vi "Get Inner Decoration.vi"() -> ()   [LabVIEW 2012] (continued)
  (unwired) 21764 items=[".NET容器"=2125, ".NET引用句柄"=3441, "10的幂"=1212, "10的自然对数"=23513, "2的幂"=1223, "2的自然对数"=23514, "ActiveX容器"=2072, "Agitator"=3831, "Array Interface Control"=23777, "Bin#1"=3073, "Bin#2"=21755, "CAN接口（程序框图常量）"=2123, "CAN接口（经典）"=3339, "CAN接口（系统）"=21964, "CAN接口（新式）"=21815, "CAN任务（程序框图常量）"=3471, "CAN任务（经典）"=3470, "CAN任务（系统）"=21963, "CAN任务（新式）"=21789, "CAN通道（程序框图常量）"=2124, "CAN通道（经典）"=3340, "CAN通道（系统）"=21966, "CAN通道（新式）"=21817, "CPU信息"=24130, "DAQmx换算名（程序框图常量）"=2116, "DAQmx换算名（经典）"=3317, "DAQmx换算名（系统）"=21952, "DAQmx换算名（新式）"=21775, "DAQmx接线端（程序框图常量）"=2117, "DAQmx接线端（经典）"=3319, "DAQmx接线端（系统）"=21955, "DAQmx接线端（新式）"=21781, "DAQmx开关（程序框图常量）"=2121, "DAQmx开关（经典）"=3337, "DAQmx开关（系统）"=21953, "DAQmx开关（新式）"=21776, "DAQmx模拟触发器源（程序框图常量）"=2119, "DAQmx模拟触发器源（经典）"=3336, "DAQmx模拟触发器源（系统）"=21951, "DAQmx模拟触发器源（新式）"=21774, "DAQmx全局通道（程序框图常量）"=3430, "DAQmx全局通道（经典）"=3443, "DAQmx全局通道（系统）"=21957, "DAQmx全局通道（新式）"=21770, "DAQmx任务名（程序框图常量）"=3434, "DAQmx任务名（经典）"=3442, "DAQmx任务名（系统）"=21959, "DAQmx任务名（新式）"=21778, "DAQmx设备名（程序框图常量）"=2093, "DAQmx设备名（经典）"=3318, "DAQmx设备名（系统）"=21950, "DAQmx设备名（新式）"=21773, "DAQmx物理通道（程序框图常量）"=2118, "DAQmx物理通道（经典）"=3335, "DAQmx物理通道（系统）"=21954, "DAQmx物理通道（新式）"=21777, "DataSocket引用句柄"=3417, "EOF"=1410, "exp(Arg)-1"=1222, "e的倒数"=23511, "FieldPoint IO点（程序框图常量）"=3440, "FieldPoint IO点（经典）"=3439, "FieldPoint IO点（新式）"=21784, "FIFO引用句柄"=3474, "For循环"=2002, "FPGA引用句柄至会话句柄转换"=2322, "Furnace"=3829, "GPIB初始化"=1957, "GPIB触发"=1953, "GPIB串行轮询"=1955, "GPIB等待"=1958, "GPIB读取"=1951, "GPIB其它命令"=1956, "GPIB清零"=1954, "GPIB写入"=1950, "GPIB状态"=1959, "IMAQ会话句柄"=3415, "IP地址至字符串转换"=1710, "IVI逻辑名称（程序框图常量）"=3420, "IVI逻辑名称（经典）"=3414, "IVI逻辑名称（新式）"=21736, "IVI删除会话句柄"=8103, "IVI新建会话句柄"=8102, "LabVIEW对象"=3457, "MathScript节点"=2357, "MATLAB脚本"=9020, "OLE变体"=3150, "Pi"=23504, "Pi乘以2"=23505, "Pi除以2"=23506, "Pi的倒数"=23507, "Pi的自然对数"=23508, "RT FIFO创建"=24000, "RT FIFO读取"=24001, "RT FIFO删除"=24003, "RT FIFO写入"=24002, "Simon量表"=32600, "Sinc"=1227, "TCP平化读取"=1718, "TCP平化写入"=1719, "TCP网络连接引用句柄"=3407, "TCP自由读取"=1720, "TCP自由写入"=1721, "TDMS Close"=24113, "TDMS Defragment"=24119, "TDMS Flush"=24117, "TDMS Get Properties"=24115, "TDMS List Contents"=24116, "TDMS Open"=24112, "TDMS Read"=24111, "TDMS Refnum To File ID"=24120, "TDMS Set Properties"=24114, "TDMS Write"=24110, "TDMS Write IP"=24118, "TDMS文件"=3477, "UDP网络连接引用句柄"=3418, "UTF-8至文本转换"=23067, "Variable Configuration"=3475, "VISA GPIB传递IFC"=2318, "VISA GPIB传递控制权"=2317, "VISA GPIB控制ATN"=2316, "VISA GPIB控制REN"=2304, "VISA GPIB命令"=2315, "VISA USB控制输出"=2087, "VISA USB控制输入"=2086, "VISA VXI命令或查询"=2305, "VISA查找资源"=1923, "VISA存数16"=1935, "VISA存数32"=1996, "VISA存数64"=2143, "VISA存数8"=1939, "VISA打开"=2308, "VISA等待事件"=1943, "VISA读取"=1925, "VISA读取STB"=1928, "VISA读取设备并写入文件"=2313, "VISA读取文件并写入设备"=2314, "VISA放弃事件"=1941, "VISA关闭"=1922, "VISA解锁"=1994, "VISA禁用事件"=1940, "VISA内存分配"=1997, "VISA内存分配Ex"=2146, "VISA内存释放"=1998, "VISA启用事件"=1942, "VISA清空I/O缓冲区"=2302, "VISA取数16"=1934, "VISA取数32"=1995, "VISA取数64"=2142, "VISA取数8"=1938, "VISA取消触发映射"=2312, "VISA取消地址映射"=1933, "VISA设备清零"=1927, "VISA设置I/O缓冲区大小"=2301, "VISA输出16"=1931, "VISA输出32"=1945, "VISA输出64"=2141, "VISA输出8"=1937, "VISA输入16"=1930, "VISA输入32"=1944, "VISA输入64"=2140, "VISA输入8"=1936, "VISA锁"=1993, "VISA写入"=1926, "VISA引用句柄至会话句柄转换"=2300, "VISA映射触发"=2311, "VISA映射地址"=1932, "VISA置触发有效"=1929, "VISA置效用信号有效"=2310, "VISA置中断信号有效"=2309, "VISA转出16"=1949, "VISA转出32"=1992, "VISA转出64"=2145, "VISA转出8"=1947, "VISA转入16"=1948, "VISA转入32"=1991, "VISA转入64"=2144, "VISA转入8"=1946, "VISA转移"=2303, "VISA状态说明"=1924, "VISA资源名称"=3421, "VISA资源名称（经典）"=3409, "VISA资源名称（新式）"=21737, "VI服务器引用"=2091, "VI库"=1425, "VI引用句柄"=3422, "While循环#1"=2003, "While循环#2"=2352, "XY图（经典）"=3500, "XY图（新式）"=21716, "X的Y次根"=23062, "X的幂"=1213, "阿伏加德罗常数(1/mol)"=23520, "按2的幂缩放"=1074, "按名称解除捆绑"=2058, "按名称捆绑"=2057, "八进制数？"=1129, "八进制字符串至数值转换"=1186, "包矩阵"=23001, "包括定点溢出状态"=5564, "保留运行类"=8018, "比特包至数组"=3135, "变量类说明符常量"=2106, "变量名称常量"=3478, "变体"=3310, "变体至平化字符串转换"=8203, "变体至数据转换"=8003, "标签（系统）"=21961, "标签（新式）"=21960, "标识符属性下拉列表"=2063, "表达式节点"=2201, "表格（经典）"=21796, "表格（系统）"=21797, "表格（新式）"=21790, "并行轮询"=1969, "并行轮询配置"=1970, "波形图（经典）"=3504, "波形图（新式）"=21703, "波形图表"=21010, "波形图表（经典）"=3501, "波形图表（新式）"=21717, "不等于0？"=1116, "不等于？"=1105, "布尔数组至数值转换"=1815, "布尔值至(0,1)转换"=1167, "步进数值控件（系统）"=21900, "彩色矩形（断开？）"=3625, "菜单下拉列表（经典）"=3018, "菜单下拉列表（新式）"=21600, "菜单引用句柄"=3413, "测试SRQ"=1986, "层叠式顺序结构"=2000, "插入菜单项"=9003, "插入式控件"=21820, "查找请求设备"=1966, "查找侦听器"=1965, "拆分按钮"=21020, "拆分路径"=1420, "拆分数字"=1170, "拆分信号"=2351, "拆分一维数组"=1908, "产生前面板活动"=1329, "产生事件发生"=1700, "产生用户定义Trace事件"=2250, "产生用户事件"=2074, "敞口槽（经典）"=3070, "敞口槽（新式）"=21751, "敞口罐（平面，经典）"=21752, "敞口罐（阴影，经典）"=3074, "乘"=1052, "乘（带错误接线端）"=3917, "程序框图禁用结构"=2054, "抽取一维数组"=2046, "初始化数组"=2053, "除"=1053, "除（带错误接线端）"=3918, "触发"=1988, "触发设备列表"=1989, "传递控制权"=1968, "传送器"=3827, "传统DAQ通道（程序框图常量）"=2085, "传统DAQ通道（经典）"=3320, "传统DAQ通道（新式）"=21733, "串行轮询所有设备"=1960, "创建TCP侦听器"=1717, "创建波形"=2066, "创建簇数组"=2047, "创建红外线侦听器"=9140, "创建矩阵"=8500, "创建蓝牙侦听器"=9151, "创建流"=23796, "创建路径"=1419, "创建数组"=2041, "创建网络流读取方端点"=23811, "创建网络流写入方端点"=23810, "创建文件夹"=8055, "创建用户事件"=2073, "垂直分隔栏"=21860, "垂直分隔栏（经典）"=21862, "垂直分隔栏（系统）"=21864, "垂直管道（平面）"=3816, "垂直管道（阴影）"=3716, "垂直滚动条"=21111, "垂直滑动杆"=3004, "垂直滑动杆（系统）"=21903, "垂直滑动杆开关（经典）"=3115, "垂直滑动杆开关（新式）"=21741, "垂直进度条（系统）"=21909, "垂直进度条（新式）"=21104, "垂直开关"=3109, "垂直刻度条"=21107, "垂直平滑盒"=3634, "垂直翘板开关"=21740, "垂直梯度矩形"=32503, "垂直梯度椭圆"=32501, "垂直梯度圆角矩形"=32506, "垂直填充滑动杆（经典）"=3009, "垂直填充滑动杆（新式）"=21014, "垂直摇杆开关（经典）"=3111, "垂直摇杆开关（新式）"=21005, "垂直直线"=3822, "垂直指针滑动杆（经典）"=3007, "垂直指针滑动杆（系统）"=21901, "垂直指针滑动杆（新式）"=21017, "从XML还原"=8401, "从流中读取单个元素"=23797, "从流中读取多个元素"=23803, "从之前设备中读取数据"=1972, "从字符串还原"=1165, "簇（经典）"=3400, "簇（新式）"=21607, "簇常量"=2071, "簇至数组转换"=1169, "错误下拉列表常量"=2039, "打开/创建/替换数据记录文件"=8054, "打开/创建/替换文件"=8050, "打开DataSocket"=1084, "打开TCP连接"=1715, "打开UDP"=1723, "打开UDP多点传送"=1727, "打开VI对象引用"=8013, "打开VI引用"=8010, "打开变量连接"=23779, "打开并验证变量连接"=23790, "打开红外线连接"=9142, "打开蓝牙连接"=9153, "打开设备"=1430, "打开文件"=1403, "打开应用程序引用"=8012, "打开自动化"=8000, "大于0？"=1117, "大于？"=1110, "大于等于0？"=1114, "大于等于？"=1103, "带边框颜色盒（经典）"=3008, "带边框颜色盒（新式）"=21019, "带标签方形按钮"=3123, "带标签矩形按钮"=3124, "带标签椭圆形按钮"=3125, "带标签圆形按钮"=3122, "带箭头线（粗）"=3631, "带箭头线（细）"=3628, "带进位的右移位"=1607, "带进位的左移位"=1606, "带阴影的椭圆"=32509, "带阴影的圆角矩形"=32508, "代码接口节点"=2050, "单按钮对话框"=1340, "单位转换"=2059, "单选按钮（经典）"=22003, "单选按钮（系统）"=22002, "单选按钮（系统） 1"=3133, "单选按钮（新式）"=22001, "弹出菜单下拉列表"=3017, "当前VI菜单栏"=9000, "当前VI路径"=1426, "当前进程ID"=24131, "倒数"=1059, "等待(ms)"=1302, "等待GPIB RQS"=1952, "等待SRQ"=1990, "等待TCP侦听器"=1712, "等待带通知器历史的多个通知"=9132, "等待带通知器历史的通知"=9131, "等待多个通知"=9106, "等待红外线侦听器"=9143, "等待活动"=1722, "等待蓝牙侦听器"=9147, "等待前面板活动"=1328, "等待事件发生"=1701, "等待通知"=9105, "等待下一个整数倍毫秒"=1327, "等于0？"=1113, "等于？"=1102, "底数为10的对数"=1210, "底数为2的对数"=1225, "底数为X的对数"=1224, "电子表格字符串至数组转换"=1539, "调用父方法"=2354, "调用节点"=3900, "调用库函数节点"=2062, "调用链"=1999, "调整矩阵大小"=8508, "定点溢出？"=5565, "定点转换为整型"=5566, "定时顺序"=5573, "定时循环"=5570, "动态FPGA接口转换"=5690, "读取DataSocket"=1086, "读取TCP数据"=1716, "读取UDP数据"=1724, "读取变量"=23781, "读取变量（超时方式）"=23786, "读取二进制文件"=8051, "读取红外线数据"=9145, "读取蓝牙数据"=9149, "读取设备"=1432, "读取数据记录文件"=8069, "读取文本文件"=8070, "读取文件"=1407, "读取状态"=1973, "队列引用句柄"=3424, "队列最前端插入元素"=9129, "对话框垂直滚动条"=21906, "对话框数值#1"=2100, "对话框数值#2"=3006, "对话框水平滚动条"=21905, "对话框字符串"=2110, "多段管道"=23780, "多列列表框（经典）"=21799, "多列列表框（系统）"=21798, "多列列表框（新式）"=21791, "多速率结构"=2199, "二维数组转置"=1902, "二维图片"=3508, "发动机（平面）"=3820, "发动机（阴影）"=3720, "发送"=1977, "发送IFC"=1980, "发送LLO"=1982, "发送命令"=1978, "发送设置"=1983, "发送数据"=1979, "发送通知"=9104, "发送至设备列表"=1981, "反馈节点"=2353, "反双曲余割"=23056, "反双曲余切"=23058, "反双曲余弦"=1218, "反双曲正割"=23057, "反双曲正切"=1219, "反双曲正弦"=1217, "反余割"=23050, "反余切"=23052, "反余弦"=1207, "反正割"=23051, "反正切"=1208, "反正切（2个输入）"=1228, "反正弦"=1206, "反转一维数组"=1900, "反转字符串"=1537, "方形按钮"=3101, "方形单选按钮"=3107, "方形灯"=3105, "方形开关按钮"=3119, "方形开关按钮（性能分析）"=3113, "方形指示灯（经典）"=3121, "方形指示灯（新式）"=21013, "访问权限"=1412, "非"=1064, "非法共享变量"=23527, "非法路径常量"=23524, "非法数字/路径/引用句柄？"=1128, "非法引用句柄常量"=23526, "分叉"=2194, "分解变体"=2404, "分解数组"=2412, "分解锁定数据变量引用"=2406, "分数/指数字符串至数值转换"=1187, "符号"=1049, "浮点数等于？"=23064, "复共轭"=1048, "复合运算"=2200, "复数至极坐标转换"=1045, "复数至实部虚部转换"=1044, "复选框（经典）"=3117, "复选框（系统）"=3132, "复选框（新式）"=21924, "复制"=8053, "复制（过时）"=1416, "负无穷大"=23509, "格式化日期/时间字符串"=8100, "格式化写入文件"=2083, "格式化写入字符串"=2081, "格式化值"=1512, "公式节点"=2004, "共享变量"=23778, "共享变量常量"=3473, "共享变量控件（经典）"=3472, "共享变量控件（新式）"=21814, "共享变量至字符串转换"=1831, "构造器节点"=3904, "关闭DataSocket"=1085, "关闭TCP连接"=1713, "关闭UDP"=1726, "关闭变量连接"=23783, "关闭红外线连接"=9144, "关闭蓝牙连接"=9148, "关闭文件"=8052, "关闭文件（过时）"=1405, "关闭引用"=8011, "关闭自动化"=8001, "合并错误"=2147, "合并信号"=2350, "红外线网络连接引用句柄"=3450, "滑动开关"=21011, "缓存级别数量"=24133, "换行符常量"=23501, "回车键常量"=23500, "回调事件引用句柄"=3435, "会话句柄至引用句柄转换"=2307, "混合复选框（系统）"=21333, "混合信号图"=21721, "获取帮助窗口状态"=1354, "获取变体属性"=8205, "获取波形成分"=2067, "获取波形属性"=8208, "获取菜单项信息"=9005, "获取定点分量"=11163, "获取队列引用"=9108, "获取队列状态"=9110, "获取记录数量"=8064, "获取矩阵对角"=8501, "获取矩阵元素"=8502, "获取卷信息"=8067, "获取快捷菜单信息"=9007, "获取权限"=8065, "获取日期/时间（秒）"=1303, "获取日期/时间字符串"=1600, "获取数据记录位置"=8061, "获取所选菜单项"=9001, "获取通知器引用"=9101, "获取通知器状态"=9103, "获取拖放数据"=9154, "获取文件大小"=8063, "获取文件类型和创建者"=8066, "获取文件位置"=8062, "获取子矩阵"=8503, "或"=1062, "或非"=1072, "基本单位转换"=1079, "极坐标至复数转换"=1047, "极坐标至实部虚部转换"=23061, "计算机ε"=23528, "加"=1050, "加1"=1057, "加（带错误接线端）"=3915, "假常量"=2006, "检查值"=3833, "简易垂直滑动杆"=3002, "简易数值"=2900, "简易水平滑动杆"=3003, "简易字符串"=2115, "减"=1051, "减1"=1058, "减（带错误接线端）"=3916, "交叉"=2197, "交换器"=3828, "交换向量元素"=1912, "交换值"=2401, "交换字"=1163, "交换字节"=1162, "交织一维数组"=2045, "接收数据"=1974, "截取字符串"=1503, "解除捆绑"=2048, "静态VI引用"=2084, "旧VISA打开"=1921, "局部变量"=2061, "矩形停止按钮"=3128, "矩阵大小"=8507, "矩阵转置"=8509, "拒绝访问"=8057, "句柄存数"=1605, "句柄取数"=1604, "卷信息"=1414, "绝对值"=1054, "开关按钮"=21001, "可打印？"=1124, "空白？"=1125, "空路径常量"=23523, "空数组？"=23063, "空字符串/路径？"=1112, "空字符串常量"=23503, "控件引用句柄"=3419, "控件与仿真循环"=2099, "控制帮助窗口"=1353, "控制在线帮助"=1355, "捆绑"=2049, "蓝牙网络连接引用句柄"=3468, "类说明符常量"=2094, "类型和创建者"=1434, "里德伯常数(1/m)"=23521, "连接"=2195, "连接字符串"=2040, "量表（经典）"=3040, "量表（新式）"=21009, "列表框（经典）"=21806, "列表框（系统）"=21805, "列表框（新式）"=21792, "列表框符号下拉列表控件常量"=2038, "列表目录"=1418, "临时目录"=1435, "漏斗#1"=21754, "漏斗#2"=3072, "路径常量"=2009, "路径类型"=1421, "路径至字符串数组转换"=1423, "路径至字符串转换"=1077, "罗列文件夹"=8083, "逻辑移位"=1081, "枚举（经典）"=3023, "枚举（系统）"=3062, "枚举（新式）"=21605, "枚举常量"=2090, "秒至日期/时间转换"=1309, "摩尔气体常数(J/(mol K))"=23522, "默认目录"=1427, "内嵌C节点"=2104, "判定范围并强制转换"=1127, "匹配模式"=1535, "匹配真/假字符串"=1533, "匹配字符串"=1532, "平方"=23059, "平方根"=1060, "平滑的椭圆"=32500, "平滑的圆角矩形"=32505, "平化至XML"=8400, "平化至字符串"=1164, "平化字符串至变体转换"=8202, "平面反向三角形"=3623, "平面方形按钮"=3103, "平面盒"=3602, "平面框"=3608, "平面右向三角形"=3621, "平面圆盒"=3611, "平面圆形"=3605, "平面圆形按钮"=3102, "平面正向三角形"=3622, "平面左向三角形"=3620, "平铺式顺序结构"=2069, "平台平面方形按钮"=3134, "普朗克常数(J/Hz)"=23516, "启用本地模式"=1963, "启用菜单跟踪"=9002, "启用远程模式"=1964, "强度图（经典）"=3510, "强度图（新式）"=21720, "强度图表（经典）"=3509, "强度图表（新式）"=21719, "强制类型转换"=1166, "强制转换至类型"=2402, "翘板开关"=21002, "清除定点溢出状态"=5562, "清空队列"=9114, "请求释放内存"=1610, "区域"=2196, "取负数"=1069, "取消按钮（系统）"=3131, "取消按钮（新式）"=21739, "取消并行轮询配置"=1971, "取消释放变体值引用"=2411, "取消通知"=9107, "取消注册会话句柄"=2320, "取消注册事件"=2076, "全局变量"=2060, "确定按钮（系统）"=3130, "确定按钮（新式）"=21738, "日期/时间至秒转换"=1308, "三维图片"=23776, "扫描变量读取"=23784, "扫描变量写入"=23787, "扫描文件"=2082, "扫描值"=1534, "扫描字符串"=2080, "删除"=8056, "删除（过时）"=1417, "删除变体属性"=8206, "删除波形属性"=8209, "删除菜单项"=9004, "删除定点溢出状态"=5563, "删除数据值引用"=2409, "删除数组元素"=3912, "商与余数"=1056, "上矩形值（轮廓）"=21762, "上矩形值（平面）"=3702, "上矩形值（阴影）"=3802, "上凸反向三角形"=3615, "上凸盒（经典）"=3600, "上凸盒（新式）"=3637, "上凸框"=3606, "上凸右向三角形"=3613, "上凸圆盒"=3609, "上凸圆形"=3603, "上凸正向三角形"=3614, "上凸左向三角形"=3612, "设备控制/状态"=1433, "设备清零"=1961, "设备清零列表"=1962, "设备引用句柄"=3405, "设置RWLS"=1984, "设置变体属性"=8204, "设置波形属性"=8207, "设置菜单项信息"=9006, "设置超时"=1985, "设置记录数量"=8075, "设置矩阵对角"=8504, "设置矩阵元素"=8505, "设置句柄大小"=1603, "设置权限"=8076, "设置事件发生"=1702, "设置数据记录位置"=8072, "设置文件大小"=8074, "设置文件类型和创建者"=8077, "设置文件位置"=8073, "设置子矩阵"=8506, "生成地址"=1967, "十进制数？"=1119, "十进制数字符串至数值转换"=1184, "十六进制数？"=1123, "十六进制数字符串至数值转换"=1185, "时间标识（程序框图常量）"=2068, "时间标识输入控件（经典）"=5555, "时间标识输入控件（系统）"=21967, "时间标识输入控件（新式）"=21913, "时间标识显示控件（经典）"=5556, "时间标识显示控件（新式）"=21914, "时间计数器"=1300, "实部虚部至复数转换"=1046, "实部虚部至极坐标转换"=23060, "事件发生引用句柄"=3406, "事件回调注册"=2078, "事件结构"=2052, "事件数据节点"=2102, "释放变体值引用"=2410, "释放队列引用"=9109, "释放通知器引用"=9102, "首次调用？"=1083, "属性节点"=1920, "树形控件（经典）"=21819, "树形控件（系统）"=21794, "树形控件（新式）"=21793, "数据缓冲区大小"=24132, "数据记录文件引用句柄"=3402, "数据值引用"=3476, "数据值引用常量"=24134, "数值常量"=2005, "数值控件（经典）"=3000, "数值控件（系统）"=21919, "数值控件（新式）"=21003, "数值显示控件（经典）"=3001, "数值显示控件（新式）"=21004, "数值至八进制字符串转换"=1182, "数值至布尔数组转换"=1814, "数值至工程字符串转换"=1183, "数值至十进制数字符串转换"=1180, "数值至十六进制字符串转换"=1181, "数值至小数字符串转换"=1506, "数值至指数字符串转换"=1505, "数字波形图（经典）"=3511, "数字波形图（新式）"=21718, "数字数据（经典）"=3210, "数字数据（新式）"=21216, "数组（程序框图常量）"=2070, "数组（经典）"=3300, "数组（新式）"=21608, "数组插入"=3911, "数组大小"=1809, "数组元素或操作"=1910, "数组元素相乘"=1904, "数组元素相加"=1903, "数组元素与操作"=1911, "数组至比特包"=3136, "数组至簇转换"=1168, "数组至电子表格字符串转换"=1540, "数组子集"=2044, "数组最大值与最小值"=1907, "刷新流"=23808, "刷新文件"=8059, "刷新文件（过时）"=1406, "双按钮对话框"=1341, "双曲余割"=23053, "双曲余切"=23055, "双曲余弦"=1215, "双曲正割"=23054, "双曲正切"=1216, "双曲正弦"=1214, "水平按钮框"=3636, "水平分隔栏"=21861, "水平分隔栏（经典）"=21863, "水平分隔栏（系统）"=21865, "水平管道（平面）"=3810, "水平管道（阴影）"=3710, "水平罐"=3071, "水平滚动条"=21110, "水平滑动杆（经典）"=3010, "水平滑动杆（系统）"=21904, "水平滑动开关"=3114, "水平进度条（系统）"=21910, "水平进度条（新式）"=21102, "水平开关"=3108, "水平刻度条"=21106, "水平平滑盒"=3633, "水平梯度矩形"=32504, "水平梯度椭圆"=32502, "水平梯度圆角矩形"=32507, "水平填充滑动杆（经典）"=3012, "水平填充滑动杆（新式）"=21100, "水平线"=3821, "水平摇杆开关（经典）"=3110, "水平摇杆开关（新式）"=21700, "水平指针滑动杆（经典）"=3011, "水平指针滑动杆（系统）"=21902, "水平指针滑动杆（新式）"=21101, "搜索"=1409, "搜索/拆分字符串"=1538, "搜索变量容器"=23802, "搜索红外线"=9141, "搜索蓝牙设备"=9152, "搜索替换字符串"=3914, "搜索一维数组"=1901, "随机数(0-1)"=1070, "索引数组"=2042, "索引与捆绑簇数组"=2056, "索引字符串数组"=1531, "锁定范围"=1411, "替换数组子集"=3910, "替换子字符串"=3913, "添加真/假字符串"=1511, "条件结构"=2001, "条件禁用结构"=2064, "停止"=1350, "停止按钮"=21230, "通过引用调用"=3901, "通过引用调用MathScript"=3906, "通知器引用句柄"=3423, "同或"=1073, "图片下拉列表（经典）"=3015, "图片下拉列表（系统）"=21925, "图片下拉列表（新式）"=21602, "退出LabVIEW"=1352, "尾数与指数"=1150, "未组合的矩阵"=23000, "温度计（经典）"=3021, "温度计（新式）"=21007, "文本按钮"=21015, "文本下拉列表（程序框图常量）"=2008, "文本下拉列表（经典）"=3014, "文本下拉列表（系统）"=3060, "文本下拉列表（新式）"=21601, "文本与图片下拉列表（经典）"=3016, "文本与图片下拉列表（新式）"=21603, "文本至UTF-8转换"=23066, "文件/目录信息"=8082, "文件/目录信息（过时）"=1413, "文件对话框"=8058, "文件对话框（过时）"=8081, "文件路径输入控件（经典）"=3203, "文件路径输入控件（系统）"=21922, "文件路径输入控件（新式）"=21730, "文件路径显示控件（经典）"=3204, "文件路径显示控件（新式）"=21731, "系统测试"=1987, "系统复位"=1976, "下凹菜单下拉列表"=3019, "下凹反向三角形"=3619, "下凹盒"=3601, "下凹盒（粗）"=3635, "下凹框（系统）"=3624, "下凹框（新式）"=3607, "下凹右向三角形"=3617, "下凹圆盒"=3610, "下凹圆盒 1"=3638, "下凹圆形"=3604, "下凹正向三角形"=3618, "下凹左向三角形"=3616, "下矩形值（轮廓）"=3806, "下矩形值（平面）"=3706, "下矩形值（阴影）"=21766, "下拉菜单下拉列表"=3061, "线条（粗）"=3629, "线条（分隔，粗）"=3630, "线条（分隔，系统）"=3632, "线条（分隔，细）"=3627, "线条（细）"=3626, "像素图"=3505, "像素图（警告：危险）"=3507, "向流中写入单个元素"=23798, "向流中写入多个元素"=23804, "向上T形（平面）"=3812, "向上T形（阴影）"=3712, "向上箭头"=3823, "向上箭头值（轮廓）"=3803, "向上箭头值（平面）"=3703, "向上箭头值（阴影）"=21763, "向上取整"=1076, "向下T形（平面）"=3818, "向下T形（阴影）"=3718, "向下箭头"=3824, "向下箭头值（轮廓）"=3807, "向下箭头值（平面）"=3707, "向下箭头值（阴影）"=21767, "向下取整"=1075, "向右T形（平面）"=3815, "向右T形（阴影）"=3715, "向左T形（平面）"=3809, "向左T形（阴影）"=3709, "向左箭头值（轮廓）"=3801, "向左箭头值（平面）"=3701, "向左箭头值（阴影）"=21761, "销毁流端点"=23794, "销毁用户事件"=2075, "小于0？"=1118, "小于？"=1111, "小于等于0？"=1115, "小于等于？"=1104, "写入DataSocket"=1087, "写入TCP数据"=1714, "写入UDP数据"=1725, "写入变量"=23782, "写入变量（超时方式）"=23789, "写入二进制文件"=8078, "写入红外线数据"=9146, "写入蓝牙数据"=9150, "写入设备"=1431, "写入数据记录文件"=8079, "写入文本文件"=8080, "写入文件"=1408, "新建VI"=8014, "新建VI对象"=8015, "新建目录"=1402, "新建数据值引用"=2408, "新文件"=1404, "行结束常量"=23525, "旋钮（经典）"=3005, "旋钮（新式）"=21000, "旋转供给器"=3830, "选项卡控件（经典）"=3330, "选项卡控件（系统）"=3331, "选项卡控件（新式）"=3332, "选行并添加至字符串"=1510, "选择"=1516, "循环移位"=1082, "压力罐（平面）"=3075, "压力罐（阴影）"=21753, "压缩器"=3832, "颜色盒"=3013, "颜色盒常量"=2120, "颜色盒窄边"=2905, "颜色梯度"=3022, "液罐（经典）"=3020, "液罐（新式）"=21006, "一维数组插值"=1905, "一维数组排序"=1120, "一维数组循环移位"=1906, "一维数组转置"=23068, "移动"=8068, "移动（过时）"=1415, "仪表（经典）"=3030, "仪表（新式）"=21008, "以10为底的e的对数"=23512, "以阈值插值一维数组"=1909, "异或"=1063, "引用句柄至会话句柄转换"=2306, "引用句柄至路径转换"=1424, "应用程序引用句柄"=3412, "用户定义标识符（程序框图常量）"=2114, "用户定义标识符（经典）"=3329, "用户定义标识符（新式）"=21749, "用户定义引用句柄"=3428, "用户定义引用句柄标识符（程序框图常量）"=3426, "用户定义引用句柄标识符（经典）"=3429, "用户定义引用句柄标识符（新式）"=21745, "用户定义引用句柄标识符平化（经典）"=3454, "用户定义引用句柄标识符平化（新式）"=21747, "用户项"=3506, "有损耗元素入队列"=9130, "右泵（平面）"=3819, "右泵（阴影）"=3719, "右箭头"=3825, "右箭头值（轮廓）"=3805, "右箭头值（平面）"=3705, "右箭头值（阴影）"=21765, "右矩形值（轮廓）"=3804, "右矩形值（平面）"=3704, "右矩形值（阴影）"=21764, "右上弯管（平面）"=3814, "右上弯管（阴影）"=3714, "右下弯管（平面）"=3817, "右下弯管（阴影）"=3717, "余割"=1204, "余切"=1205, "余弦"=1201, "与"=1061, "与非"=1071, "预分配的读取二进制文件"=24135, "预览队列元素"=9112, "元电荷(C)"=23517, "元素出队列"=9113, "元素入队列"=9111, "元素同址操作结构"=2360, "圆形按钮"=3100, "圆形单选按钮"=3106, "圆形灯"=3104, "圆形开关按钮"=3118, "圆形开关按钮（性能分析）"=3112, "圆形停止按钮"=3127, "圆形指示灯（经典）"=3120, "圆形指示灯（新式）"=21012, "运动资源（程序框图常量）"=3449, "运动资源（经典）"=3448, "运动资源（新式）"=21787, "蕴含"=1080, "在后台打开变量连接"=23791, "在字符串中搜索标记"=8101, "真空光速(m/sec)"=23518, "整数拼接"=1171, "整型转换为定点"=5567, "正割"=1203, "正切"=1202, "正无穷大"=23515, "正弦"=1200, "正弦与余弦"=1220, "直接变量读取"=23785, "直接变量写入"=23788, "指示灯按钮"=3116, "指数"=1211, "制表符常量"=23502, "重力常数(Nm2/kg2)"=23519, "重排数组维数"=2055, "重组变体（警告：危险）"=2405, "重组解锁数据变量引用（警告：危险）"=2407, "重组数组"=2403, "注册会话句柄"=2319, "注册事件"=2065, "转换为64位整型"=1155, "转换为OLE变体"=8002, "转换为变体"=8201, "转换为长整型"=1142, "转换为大写字母"=1188, "转换为单精度浮点数"=1146, "转换为单精度复数"=1151, "转换为单字节整型"=1140, "转换为定点数"=5561, "转换为扩展精度浮点数"=1149, "转换为扩展精度复数"=1154, "转换为时间标识"=5560, "转换为双精度浮点数"=1147, "转换为双精度复数"=1152, "转换为双字节整型"=1141, "转换为探针字符串"=2413, "转换为特定的类"=8016, "转换为通用的类"=8017, "转换为无符号64位整型"=1156, "转换为无符号长整型"=1145, "转换为无符号单字节整型"=1143, "转换为无符号双字节整型"=1144, "转换为小写字母"=1189, "转盘（经典）"=3050, "转盘（新式）"=21732, "状态"=2198, "状态图"=2051, "准备接收"=1975, "资源索引"=1088, "子面板"=21810, "子面板（经典）"=21811, "子面板（系统）"=21823, "自动化引用句柄"=3410, "自然对数"=1209, "自然对数 (Arg +1)"=1221, "自然对数的底数"=23510, "自由标签"=2321, "字符串常量"=2007, "字符串长度"=1502, "字符串输入控件（经典）"=3200, "字符串输入控件（系统）"=21920, "字符串输入控件（新式）"=21701, "字符串数组排序"=23065, "字符串数组至路径转换"=1422, "字符串显示控件（经典）"=3201, "字符串显示控件（新式）"=21702, "字符串移位"=1536, "字符串至IP地址转换"=1711, "字符串至共享变量转换"=1830, "字符串至路径转换"=1078, "字符串至字节数组转换"=1608, "字符类"=1126, "字节流文件引用句柄"=3408, "字节数组至字符串转换"=1609, "总是复制"=2400, "组合框（经典）"=3304, "组合框（系统）"=21917, "组合框（新式）"=21604, "组合框常量"=2088, "最大值与最小值"=1108, "最近数取整"=1055, "左泵（平面）"=3813, "左泵（阴影）"=3713, "左箭头"=3826, "左矩形值（轮廓）"=3800, "左矩形值（平面）"=3700, "左矩形值（阴影）"=21760, "左上弯管（平面）"=3808, "左上弯管（阴影）"=3708, "左下弯管（平面）"=3811, "左下弯管（阴影）"=3711]
  (unwired) 21764 items=[".NET容器"=2125, ".NET引用句柄"=3441, "10的幂"=1212, "10的自然对数"=23513, "2的幂"=1223, "2的自然对数"=23514, "ActiveX容器"=2072, "Agitator"=3831, "Array Interface Control"=23777, "Bin#1"=3073, "Bin#2"=21755, "CAN接口（程序框图常量）"=2123, "CAN接口（经典）"=3339, "CAN接口（系统）"=21964, "CAN接口（新式）"=21815, "CAN任务（程序框图常量）"=3471, "CAN任务（经典）"=3470, "CAN任务（系统）"=21963, "CAN任务（新式）"=21789, "CAN通道（程序框图常量）"=2124, "CAN通道（经典）"=3340, "CAN通道（系统）"=21966, "CAN通道（新式）"=21817, "CPU信息"=24130, "DAQmx换算名（程序框图常量）"=2116, "DAQmx换算名（经典）"=3317, "DAQmx换算名（系统）"=21952, "DAQmx换算名（新式）"=21775, "DAQmx接线端（程序框图常量）"=2117, "DAQmx接线端（经典）"=3319, "DAQmx接线端（系统）"=21955, "DAQmx接线端（新式）"=21781, "DAQmx开关（程序框图常量）"=2121, "DAQmx开关（经典）"=3337, "DAQmx开关（系统）"=21953, "DAQmx开关（新式）"=21776, "DAQmx模拟触发器源（程序框图常量）"=2119, "DAQmx模拟触发器源（经典）"=3336, "DAQmx模拟触发器源（系统）"=21951, "DAQmx模拟触发器源（新式）"=21774, "DAQmx全局通道（程序框图常量）"=3430, "DAQmx全局通道（经典）"=3443, "DAQmx全局通道（系统）"=21957, "DAQmx全局通道（新式）"=21770, "DAQmx任务名（程序框图常量）"=3434, "DAQmx任务名（经典）"=3442, "DAQmx任务名（系统）"=21959, "DAQmx任务名（新式）"=21778, "DAQmx设备名（程序框图常量）"=2093, "DAQmx设备名（经典）"=3318, "DAQmx设备名（系统）"=21950, "DAQmx设备名（新式）"=21773, "DAQmx物理通道（程序框图常量）"=2118, "DAQmx物理通道（经典）"=3335, "DAQmx物理通道（系统）"=21954, "DAQmx物理通道（新式）"=21777, "DataSocket引用句柄"=3417, "EOF"=1410, "exp(Arg)-1"=1222, "e的倒数"=23511, "FieldPoint IO点（程序框图常量）"=3440, "FieldPoint IO点（经典）"=3439, "FieldPoint IO点（新式）"=21784, "FIFO引用句柄"=3474, "For循环"=2002, "FPGA引用句柄至会话句柄转换"=2322, "Furnace"=3829, "GPIB初始化"=1957, "GPIB触发"=1953, "GPIB串行轮询"=1955, "GPIB等待"=1958, "GPIB读取"=1951, "GPIB其它命令"=1956, "GPIB清零"=1954, "GPIB写入"=1950, "GPIB状态"=1959, "IMAQ会话句柄"=3415, "IP地址至字符串转换"=1710, "IVI逻辑名称（程序框图常量）"=3420, "IVI逻辑名称（经典）"=3414, "IVI逻辑名称（新式）"=21736, "IVI删除会话句柄"=8103, "IVI新建会话句柄"=8102, "LabVIEW对象"=3457, "MathScript节点"=2357, "MATLAB脚本"=9020, "OLE变体"=3150, "Pi"=23504, "Pi乘以2"=23505, "Pi除以2"=23506, "Pi的倒数"=23507, "Pi的自然对数"=23508, "RT FIFO创建"=24000, "RT FIFO读取"=24001, "RT FIFO删除"=24003, "RT FIFO写入"=24002, "Simon量表"=32600, "Sinc"=1227, "TCP平化读取"=1718, "TCP平化写入"=1719, "TCP网络连接引用句柄"=3407, "TCP自由读取"=1720, "TCP自由写入"=1721, "TDMS Close"=24113, "TDMS Defragment"=24119, "TDMS Flush"=24117, "TDMS Get Properties"=24115, "TDMS List Contents"=24116, "TDMS Open"=24112, "TDMS Read"=24111, "TDMS Refnum To File ID"=24120, "TDMS Set Properties"=24114, "TDMS Write"=24110, "TDMS Write IP"=24118, "TDMS文件"=3477, "UDP网络连接引用句柄"=3418, "UTF-8至文本转换"=23067, "Variable Configuration"=3475, "VISA GPIB传递IFC"=2318, "VISA GPIB传递控制权"=2317, "VISA GPIB控制ATN"=2316, "VISA GPIB控制REN"=2304, "VISA GPIB命令"=2315, "VISA USB控制输出"=2087, "VISA USB控制输入"=2086, "VISA VXI命令或查询"=2305, "VISA查找资源"=1923, "VISA存数16"=1935, "VISA存数32"=1996, "VISA存数64"=2143, "VISA存数8"=1939, "VISA打开"=2308, "VISA等待事件"=1943, "VISA读取"=1925, "VISA读取STB"=1928, "VISA读取设备并写入文件"=2313, "VISA读取文件并写入设备"=2314, "VISA放弃事件"=1941, "VISA关闭"=1922, "VISA解锁"=1994, "VISA禁用事件"=1940, "VISA内存分配"=1997, "VISA内存分配Ex"=2146, "VISA内存释放"=1998, "VISA启用事件"=1942, "VISA清空I/O缓冲区"=2302, "VISA取数16"=1934, "VISA取数32"=1995, "VISA取数64"=2142, "VISA取数8"=1938, "VISA取消触发映射"=2312, "VISA取消地址映射"=1933, "VISA设备清零"=1927, "VISA设置I/O缓冲区大小"=2301, "VISA输出16"=1931, "VISA输出32"=1945, "VISA输出64"=2141, "VISA输出8"=1937, "VISA输入16"=1930, "VISA输入32"=1944, "VISA输入64"=2140, "VISA输入8"=1936, "VISA锁"=1993, "VISA写入"=1926, "VISA引用句柄至会话句柄转换"=2300, "VISA映射触发"=2311, "VISA映射地址"=1932, "VISA置触发有效"=1929, "VISA置效用信号有效"=2310, "VISA置中断信号有效"=2309, "VISA转出16"=1949, "VISA转出32"=1992, "VISA转出64"=2145, "VISA转出8"=1947, "VISA转入16"=1948, "VISA转入32"=1991, "VISA转入64"=2144, "VISA转入8"=1946, "VISA转移"=2303, "VISA状态说明"=1924, "VISA资源名称"=3421, "VISA资源名称（经典）"=3409, "VISA资源名称（新式）"=21737, "VI服务器引用"=2091, "VI库"=1425, "VI引用句柄"=3422, "While循环#1"=2003, "While循环#2"=2352, "XY图（经典）"=3500, "XY图（新式）"=21716, "X的Y次根"=23062, "X的幂"=1213, "阿伏加德罗常数(1/mol)"=23520, "按2的幂缩放"=1074, "按名称解除捆绑"=2058, "按名称捆绑"=2057, "八进制数？"=1129, "八进制字符串至数值转换"=1186, "包矩阵"=23001, "包括定点溢出状态"=5564, "保留运行类"=8018, "比特包至数组"=3135, "变量类说明符常量"=2106, "变量名称常量"=3478, "变体"=3310, "变体至平化字符串转换"=8203, "变体至数据转换"=8003, "标签（系统）"=21961, "标签（新式）"=21960, "标识符属性下拉列表"=2063, "表达式节点"=2201, "表格（经典）"=21796, "表格（系统）"=21797, "表格（新式）"=21790, "并行轮询"=1969, "并行轮询配置"=1970, "波形图（经典）"=3504, "波形图（新式）"=21703, "波形图表"=21010, "波形图表（经典）"=3501, "波形图表（新式）"=21717, "不等于0？"=1116, "不等于？"=1105, "布尔数组至数值转换"=1815, "布尔值至(0,1)转换"=1167, "步进数值控件（系统）"=21900, "彩色矩形（断开？）"=3625, "菜单下拉列表（经典）"=3018, "菜单下拉列表（新式）"=21600, "菜单引用句柄"=3413, "测试SRQ"=1986, "层叠式顺序结构"=2000, "插入菜单项"=9003, "插入式控件"=21820, "查找请求设备"=1966, "查找侦听器"=1965, "拆分按钮"=21020, "拆分路径"=1420, "拆分数字"=1170, "拆分信号"=2351, "拆分一维数组"=1908, "产生前面板活动"=1329, "产生事件发生"=1700, "产生用户定义Trace事件"=2250, "产生用户事件"=2074, "敞口槽（经典）"=3070, "敞口槽（新式）"=21751, "敞口罐（平面，经典）"=21752, "敞口罐（阴影，经典）"=3074, "乘"=1052, "乘（带错误接线端）"=3917, "程序框图禁用结构"=2054, "抽取一维数组"=2046, "初始化数组"=2053, "除"=1053, "除（带错误接线端）"=3918, "触发"=1988, "触发设备列表"=1989, "传递控制权"=1968, "传送器"=3827, "传统DAQ通道（程序框图常量）"=2085, "传统DAQ通道（经典）"=3320, "传统DAQ通道（新式）"=21733, "串行轮询所有设备"=1960, "创建TCP侦听器"=1717, "创建波形"=2066, "创建簇数组"=2047, "创建红外线侦听器"=9140, "创建矩阵"=8500, "创建蓝牙侦听器"=9151, "创建流"=23796, "创建路径"=1419, "创建数组"=2041, "创建网络流读取方端点"=23811, "创建网络流写入方端点"=23810, "创建文件夹"=8055, "创建用户事件"=2073, "垂直分隔栏"=21860, "垂直分隔栏（经典）"=21862, "垂直分隔栏（系统）"=21864, "垂直管道（平面）"=3816, "垂直管道（阴影）"=3716, "垂直滚动条"=21111, "垂直滑动杆"=3004, "垂直滑动杆（系统）"=21903, "垂直滑动杆开关（经典）"=3115, "垂直滑动杆开关（新式）"=21741, "垂直进度条（系统）"=21909, "垂直进度条（新式）"=21104, "垂直开关"=3109, "垂直刻度条"=21107, "垂直平滑盒"=3634, "垂直翘板开关"=21740, "垂直梯度矩形"=32503, "垂直梯度椭圆"=32501, "垂直梯度圆角矩形"=32506, "垂直填充滑动杆（经典）"=3009, "垂直填充滑动杆（新式）"=21014, "垂直摇杆开关（经典）"=3111, "垂直摇杆开关（新式）"=21005, "垂直直线"=3822, "垂直指针滑动杆（经典）"=3007, "垂直指针滑动杆（系统）"=21901, "垂直指针滑动杆（新式）"=21017, "从XML还原"=8401, "从流中读取单个元素"=23797, "从流中读取多个元素"=23803, "从之前设备中读取数据"=1972, "从字符串还原"=1165, "簇（经典）"=3400, "簇（新式）"=21607, "簇常量"=2071, "簇至数组转换"=1169, "错误下拉列表常量"=2039, "打开/创建/替换数据记录文件"=8054, "打开/创建/替换文件"=8050, "打开DataSocket"=1084, "打开TCP连接"=1715, "打开UDP"=1723, "打开UDP多点传送"=1727, "打开VI对象引用"=8013, "打开VI引用"=8010, "打开变量连接"=23779, "打开并验证变量连接"=23790, "打开红外线连接"=9142, "打开蓝牙连接"=9153, "打开设备"=1430, "打开文件"=1403, "打开应用程序引用"=8012, "打开自动化"=8000, "大于0？"=1117, "大于？"=1110, "大于等于0？"=1114, "大于等于？"=1103, "带边框颜色盒（经典）"=3008, "带边框颜色盒（新式）"=21019, "带标签方形按钮"=3123, "带标签矩形按钮"=3124, "带标签椭圆形按钮"=3125, "带标签圆形按钮"=3122, "带箭头线（粗）"=3631, "带箭头线（细）"=3628, "带进位的右移位"=1607, "带进位的左移位"=1606, "带阴影的椭圆"=32509, "带阴影的圆角矩形"=32508, "代码接口节点"=2050, "单按钮对话框"=1340, "单位转换"=2059, "单选按钮（经典）"=22003, "单选按钮（系统）"=22002, "单选按钮（系统） 1"=3133, "单选按钮（新式）"=22001, "弹出菜单下拉列表"=3017, "当前VI菜单栏"=9000, "当前VI路径"=1426, "当前进程ID"=24131, "倒数"=1059, "等待(ms)"=1302, "等待GPIB RQS"=1952, "等待SRQ"=1990, "等待TCP侦听器"=1712, "等待带通知器历史的多个通知"=9132, "等待带通知器历史的通知"=9131, "等待多个通知"=9106, "等待红外线侦听器"=9143, "等待活动"=1722, "等待蓝牙侦听器"=9147, "等待前面板活动"=1328, "等待事件发生"=1701, "等待通知"=9105, "等待下一个整数倍毫秒"=1327, "等于0？"=1113, "等于？"=1102, "底数为10的对数"=1210, "底数为2的对数"=1225, "底数为X的对数"=1224, "电子表格字符串至数组转换"=1539, "调用父方法"=2354, "调用节点"=3900, "调用库函数节点"=2062, "调用链"=1999, "调整矩阵大小"=8508, "定点溢出？"=5565, "定点转换为整型"=5566, "定时顺序"=5573, "定时循环"=5570, "动态FPGA接口转换"=5690, "读取DataSocket"=1086, "读取TCP数据"=1716, "读取UDP数据"=1724, "读取变量"=23781, "读取变量（超时方式）"=23786, "读取二进制文件"=8051, "读取红外线数据"=9145, "读取蓝牙数据"=9149, "读取设备"=1432, "读取数据记录文件"=8069, "读取文本文件"=8070, "读取文件"=1407, "读取状态"=1973, "队列引用句柄"=3424, "队列最前端插入元素"=9129, "对话框垂直滚动条"=21906, "对话框数值#1"=2100, "对话框数值#2"=3006, "对话框水平滚动条"=21905, "对话框字符串"=2110, "多段管道"=23780, "多列列表框（经典）"=21799, "多列列表框（系统）"=21798, "多列列表框（新式）"=21791, "多速率结构"=2199, "二维数组转置"=1902, "二维图片"=3508, "发动机（平面）"=3820, "发动机（阴影）"=3720, "发送"=1977, "发送IFC"=1980, "发送LLO"=1982, "发送命令"=1978, "发送设置"=1983, "发送数据"=1979, "发送通知"=9104, "发送至设备列表"=1981, "反馈节点"=2353, "反双曲余割"=23056, "反双曲余切"=23058, "反双曲余弦"=1218, "反双曲正割"=23057, "反双曲正切"=1219, "反双曲正弦"=1217, "反余割"=23050, "反余切"=23052, "反余弦"=1207, "反正割"=23051, "反正切"=1208, "反正切（2个输入）"=1228, "反正弦"=1206, "反转一维数组"=1900, "反转字符串"=1537, "方形按钮"=3101, "方形单选按钮"=3107, "方形灯"=3105, "方形开关按钮"=3119, "方形开关按钮（性能分析）"=3113, "方形指示灯（经典）"=3121, "方形指示灯（新式）"=21013, "访问权限"=1412, "非"=1064, "非法共享变量"=23527, "非法路径常量"=23524, "非法数字/路径/引用句柄？"=1128, "非法引用句柄常量"=23526, "分叉"=2194, "分解变体"=2404, "分解数组"=2412, "分解锁定数据变量引用"=2406, "分数/指数字符串至数值转换"=1187, "符号"=1049, "浮点数等于？"=23064, "复共轭"=1048, "复合运算"=2200, "复数至极坐标转换"=1045, "复数至实部虚部转换"=1044, "复选框（经典）"=3117, "复选框（系统）"=3132, "复选框（新式）"=21924, "复制"=8053, "复制（过时）"=1416, "负无穷大"=23509, "格式化日期/时间字符串"=8100, "格式化写入文件"=2083, "格式化写入字符串"=2081, "格式化值"=1512, "公式节点"=2004, "共享变量"=23778, "共享变量常量"=3473, "共享变量控件（经典）"=3472, "共享变量控件（新式）"=21814, "共享变量至字符串转换"=1831, "构造器节点"=3904, "关闭DataSocket"=1085, "关闭TCP连接"=1713, "关闭UDP"=1726, "关闭变量连接"=23783, "关闭红外线连接"=9144, "关闭蓝牙连接"=9148, "关闭文件"=8052, "关闭文件（过时）"=1405, "关闭引用"=8011, "关闭自动化"=8001, "合并错误"=2147, "合并信号"=2350, "红外线网络连接引用句柄"=3450, "滑动开关"=21011, "缓存级别数量"=24133, "换行符常量"=23501, "回车键常量"=23500, "回调事件引用句柄"=3435, "会话句柄至引用句柄转换"=2307, "混合复选框（系统）"=21333, "混合信号图"=21721, "获取帮助窗口状态"=1354, "获取变体属性"=8205, "获取波形成分"=2067, "获取波形属性"=8208, "获取菜单项信息"=9005, "获取定点分量"=11163, "获取队列引用"=9108, "获取队列状态"=9110, "获取记录数量"=8064, "获取矩阵对角"=8501, "获取矩阵元素"=8502, "获取卷信息"=8067, "获取快捷菜单信息"=9007, "获取权限"=8065, "获取日期/时间（秒）"=1303, "获取日期/时间字符串"=1600, "获取数据记录位置"=8061, "获取所选菜单项"=9001, "获取通知器引用"=9101, "获取通知器状态"=9103, "获取拖放数据"=9154, "获取文件大小"=8063, "获取文件类型和创建者"=8066, "获取文件位置"=8062, "获取子矩阵"=8503, "或"=1062, "或非"=1072, "基本单位转换"=1079, "极坐标至复数转换"=1047, "极坐标至实部虚部转换"=23061, "计算机ε"=23528, "加"=1050, "加1"=1057, "加（带错误接线端）"=3915, "假常量"=2006, "检查值"=3833, "简易垂直滑动杆"=3002, "简易数值"=2900, "简易水平滑动杆"=3003, "简易字符串"=2115, "减"=1051, "减1"=1058, "减（带错误接线端）"=3916, "交叉"=2197, "交换器"=3828, "交换向量元素"=1912, "交换值"=2401, "交换字"=1163, "交换字节"=1162, "交织一维数组"=2045, "接收数据"=1974, "截取字符串"=1503, "解除捆绑"=2048, "静态VI引用"=2084, "旧VISA打开"=1921, "局部变量"=2061, "矩形停止按钮"=3128, "矩阵大小"=8507, "矩阵转置"=8509, "拒绝访问"=8057, "句柄存数"=1605, "句柄取数"=1604, "卷信息"=1414, "绝对值"=1054, "开关按钮"=21001, "可打印？"=1124, "空白？"=1125, "空路径常量"=23523, "空数组？"=23063, "空字符串/路径？"=1112, "空字符串常量"=23503, "控件引用句柄"=3419, "控件与仿真循环"=2099, "控制帮助窗口"=1353, "控制在线帮助"=1355, "捆绑"=2049, "蓝牙网络连接引用句柄"=3468, "类说明符常量"=2094, "类型和创建者"=1434, "里德伯常数(1/m)"=23521, "连接"=2195, "连接字符串"=2040, "量表（经典）"=3040, "量表（新式）"=21009, "列表框（经典）"=21806, "列表框（系统）"=21805, "列表框（新式）"=21792, "列表框符号下拉列表控件常量"=2038, "列表目录"=1418, "临时目录"=1435, "漏斗#1"=21754, "漏斗#2"=3072, "路径常量"=2009, "路径类型"=1421, "路径至字符串数组转换"=1423, "路径至字符串转换"=1077, "罗列文件夹"=8083, "逻辑移位"=1081, "枚举（经典）"=3023, "枚举（系统）"=3062, "枚举（新式）"=21605, "枚举常量"=2090, "秒至日期/时间转换"=1309, "摩尔气体常数(J/(mol K))"=23522, "默认目录"=1427, "内嵌C节点"=2104, "判定范围并强制转换"=1127, "匹配模式"=1535, "匹配真/假字符串"=1533, "匹配字符串"=1532, "平方"=23059, "平方根"=1060, "平滑的椭圆"=32500, "平滑的圆角矩形"=32505, "平化至XML"=8400, "平化至字符串"=1164, "平化字符串至变体转换"=8202, "平面反向三角形"=3623, "平面方形按钮"=3103, "平面盒"=3602, "平面框"=3608, "平面右向三角形"=3621, "平面圆盒"=3611, "平面圆形"=3605, "平面圆形按钮"=3102, "平面正向三角形"=3622, "平面左向三角形"=3620, "平铺式顺序结构"=2069, "平台平面方形按钮"=3134, "普朗克常数(J/Hz)"=23516, "启用本地模式"=1963, "启用菜单跟踪"=9002, "启用远程模式"=1964, "强度图（经典）"=3510, "强度图（新式）"=21720, "强度图表（经典）"=3509, "强度图表（新式）"=21719, "强制类型转换"=1166, "强制转换至类型"=2402, "翘板开关"=21002, "清除定点溢出状态"=5562, "清空队列"=9114, "请求释放内存"=1610, "区域"=2196, "取负数"=1069, "取消按钮（系统）"=3131, "取消按钮（新式）"=21739, "取消并行轮询配置"=1971, "取消释放变体值引用"=2411, "取消通知"=9107, "取消注册会话句柄"=2320, "取消注册事件"=2076, "全局变量"=2060, "确定按钮（系统）"=3130, "确定按钮（新式）"=21738, "日期/时间至秒转换"=1308, "三维图片"=23776, "扫描变量读取"=23784, "扫描变量写入"=23787, "扫描文件"=2082, "扫描值"=1534, "扫描字符串"=2080, "删除"=8056, "删除（过时）"=1417, "删除变体属性"=8206, "删除波形属性"=8209, "删除菜单项"=9004, "删除定点溢出状态"=5563, "删除数据值引用"=2409, "删除数组元素"=3912, "商与余数"=1056, "上矩形值（轮廓）"=21762, "上矩形值（平面）"=3702, "上矩形值（阴影）"=3802, "上凸反向三角形"=3615, "上凸盒（经典）"=3600, "上凸盒（新式）"=3637, "上凸框"=3606, "上凸右向三角形"=3613, "上凸圆盒"=3609, "上凸圆形"=3603, "上凸正向三角形"=3614, "上凸左向三角形"=3612, "设备控制/状态"=1433, "设备清零"=1961, "设备清零列表"=1962, "设备引用句柄"=3405, "设置RWLS"=1984, "设置变体属性"=8204, "设置波形属性"=8207, "设置菜单项信息"=9006, "设置超时"=1985, "设置记录数量"=8075, "设置矩阵对角"=8504, "设置矩阵元素"=8505, "设置句柄大小"=1603, "设置权限"=8076, "设置事件发生"=1702, "设置数据记录位置"=8072, "设置文件大小"=8074, "设置文件类型和创建者"=8077, "设置文件位置"=8073, "设置子矩阵"=8506, "生成地址"=1967, "十进制数？"=1119, "十进制数字符串至数值转换"=1184, "十六进制数？"=1123, "十六进制数字符串至数值转换"=1185, "时间标识（程序框图常量）"=2068, "时间标识输入控件（经典）"=5555, "时间标识输入控件（系统）"=21967, "时间标识输入控件（新式）"=21913, "时间标识显示控件（经典）"=5556, "时间标识显示控件（新式）"=21914, "时间计数器"=1300, "实部虚部至复数转换"=1046, "实部虚部至极坐标转换"=23060, "事件发生引用句柄"=3406, "事件回调注册"=2078, "事件结构"=2052, "事件数据节点"=2102, "释放变体值引用"=2410, "释放队列引用"=9109, "释放通知器引用"=9102, "首次调用？"=1083, "属性节点"=1920, "树形控件（经典）"=21819, "树形控件（系统）"=21794, "树形控件（新式）"=21793, "数据缓冲区大小"=24132, "数据记录文件引用句柄"=3402, "数据值引用"=3476, "数据值引用常量"=24134, "数值常量"=2005, "数值控件（经典）"=3000, "数值控件（系统）"=21919, "数值控件（新式）"=21003, "数值显示控件（经典）"=3001, "数值显示控件（新式）"=21004, "数值至八进制字符串转换"=1182, "数值至布尔数组转换"=1814, "数值至工程字符串转换"=1183, "数值至十进制数字符串转换"=1180, "数值至十六进制字符串转换"=1181, "数值至小数字符串转换"=1506, "数值至指数字符串转换"=1505, "数字波形图（经典）"=3511, "数字波形图（新式）"=21718, "数字数据（经典）"=3210, "数字数据（新式）"=21216, "数组（程序框图常量）"=2070, "数组（经典）"=3300, "数组（新式）"=21608, "数组插入"=3911, "数组大小"=1809, "数组元素或操作"=1910, "数组元素相乘"=1904, "数组元素相加"=1903, "数组元素与操作"=1911, "数组至比特包"=3136, "数组至簇转换"=1168, "数组至电子表格字符串转换"=1540, "数组子集"=2044, "数组最大值与最小值"=1907, "刷新流"=23808, "刷新文件"=8059, "刷新文件（过时）"=1406, "双按钮对话框"=1341, "双曲余割"=23053, "双曲余切"=23055, "双曲余弦"=1215, "双曲正割"=23054, "双曲正切"=1216, "双曲正弦"=1214, "水平按钮框"=3636, "水平分隔栏"=21861, "水平分隔栏（经典）"=21863, "水平分隔栏（系统）"=21865, "水平管道（平面）"=3810, "水平管道（阴影）"=3710, "水平罐"=3071, "水平滚动条"=21110, "水平滑动杆（经典）"=3010, "水平滑动杆（系统）"=21904, "水平滑动开关"=3114, "水平进度条（系统）"=21910, "水平进度条（新式）"=21102, "水平开关"=3108, "水平刻度条"=21106, "水平平滑盒"=3633, "水平梯度矩形"=32504, "水平梯度椭圆"=32502, "水平梯度圆角矩形"=32507, "水平填充滑动杆（经典）"=3012, "水平填充滑动杆（新式）"=21100, "水平线"=3821, "水平摇杆开关（经典）"=3110, "水平摇杆开关（新式）"=21700, "水平指针滑动杆（经典）"=3011, "水平指针滑动杆（系统）"=21902, "水平指针滑动杆（新式）"=21101, "搜索"=1409, "搜索/拆分字符串"=1538, "搜索变量容器"=23802, "搜索红外线"=9141, "搜索蓝牙设备"=9152, "搜索替换字符串"=3914, "搜索一维数组"=1901, "随机数(0-1)"=1070, "索引数组"=2042, "索引与捆绑簇数组"=2056, "索引字符串数组"=1531, "锁定范围"=1411, "替换数组子集"=3910, "替换子字符串"=3913, "添加真/假字符串"=1511, "条件结构"=2001, "条件禁用结构"=2064, "停止"=1350, "停止按钮"=21230, "通过引用调用"=3901, "通过引用调用MathScript"=3906, "通知器引用句柄"=3423, "同或"=1073, "图片下拉列表（经典）"=3015, "图片下拉列表（系统）"=21925, "图片下拉列表（新式）"=21602, "退出LabVIEW"=1352, "尾数与指数"=1150, "未组合的矩阵"=23000, "温度计（经典）"=3021, "温度计（新式）"=21007, "文本按钮"=21015, "文本下拉列表（程序框图常量）"=2008, "文本下拉列表（经典）"=3014, "文本下拉列表（系统）"=3060, "文本下拉列表（新式）"=21601, "文本与图片下拉列表（经典）"=3016, "文本与图片下拉列表（新式）"=21603, "文本至UTF-8转换"=23066, "文件/目录信息"=8082, "文件/目录信息（过时）"=1413, "文件对话框"=8058, "文件对话框（过时）"=8081, "文件路径输入控件（经典）"=3203, "文件路径输入控件（系统）"=21922, "文件路径输入控件（新式）"=21730, "文件路径显示控件（经典）"=3204, "文件路径显示控件（新式）"=21731, "系统测试"=1987, "系统复位"=1976, "下凹菜单下拉列表"=3019, "下凹反向三角形"=3619, "下凹盒"=3601, "下凹盒（粗）"=3635, "下凹框（系统）"=3624, "下凹框（新式）"=3607, "下凹右向三角形"=3617, "下凹圆盒"=3610, "下凹圆盒 1"=3638, "下凹圆形"=3604, "下凹正向三角形"=3618, "下凹左向三角形"=3616, "下矩形值（轮廓）"=3806, "下矩形值（平面）"=3706, "下矩形值（阴影）"=21766, "下拉菜单下拉列表"=3061, "线条（粗）"=3629, "线条（分隔，粗）"=3630, "线条（分隔，系统）"=3632, "线条（分隔，细）"=3627, "线条（细）"=3626, "像素图"=3505, "像素图（警告：危险）"=3507, "向流中写入单个元素"=23798, "向流中写入多个元素"=23804, "向上T形（平面）"=3812, "向上T形（阴影）"=3712, "向上箭头"=3823, "向上箭头值（轮廓）"=3803, "向上箭头值（平面）"=3703, "向上箭头值（阴影）"=21763, "向上取整"=1076, "向下T形（平面）"=3818, "向下T形（阴影）"=3718, "向下箭头"=3824, "向下箭头值（轮廓）"=3807, "向下箭头值（平面）"=3707, "向下箭头值（阴影）"=21767, "向下取整"=1075, "向右T形（平面）"=3815, "向右T形（阴影）"=3715, "向左T形（平面）"=3809, "向左T形（阴影）"=3709, "向左箭头值（轮廓）"=3801, "向左箭头值（平面）"=3701, "向左箭头值（阴影）"=21761, "销毁流端点"=23794, "销毁用户事件"=2075, "小于0？"=1118, "小于？"=1111, "小于等于0？"=1115, "小于等于？"=1104, "写入DataSocket"=1087, "写入TCP数据"=1714, "写入UDP数据"=1725, "写入变量"=23782, "写入变量（超时方式）"=23789, "写入二进制文件"=8078, "写入红外线数据"=9146, "写入蓝牙数据"=9150, "写入设备"=1431, "写入数据记录文件"=8079, "写入文本文件"=8080, "写入文件"=1408, "新建VI"=8014, "新建VI对象"=8015, "新建目录"=1402, "新建数据值引用"=2408, "新文件"=1404, "行结束常量"=23525, "旋钮（经典）"=3005, "旋钮（新式）"=21000, "旋转供给器"=3830, "选项卡控件（经典）"=3330, "选项卡控件（系统）"=3331, "选项卡控件（新式）"=3332, "选行并添加至字符串"=1510, "选择"=1516, "循环移位"=1082, "压力罐（平面）"=3075, "压力罐（阴影）"=21753, "压缩器"=3832, "颜色盒"=3013, "颜色盒常量"=2120, "颜色盒窄边"=2905, "颜色梯度"=3022, "液罐（经典）"=3020, "液罐（新式）"=21006, "一维数组插值"=1905, "一维数组排序"=1120, "一维数组循环移位"=1906, "一维数组转置"=23068, "移动"=8068, "移动（过时）"=1415, "仪表（经典）"=3030, "仪表（新式）"=21008, "以10为底的e的对数"=23512, "以阈值插值一维数组"=1909, "异或"=1063, "引用句柄至会话句柄转换"=2306, "引用句柄至路径转换"=1424, "应用程序引用句柄"=3412, "用户定义标识符（程序框图常量）"=2114, "用户定义标识符（经典）"=3329, "用户定义标识符（新式）"=21749, "用户定义引用句柄"=3428, "用户定义引用句柄标识符（程序框图常量）"=3426, "用户定义引用句柄标识符（经典）"=3429, "用户定义引用句柄标识符（新式）"=21745, "用户定义引用句柄标识符平化（经典）"=3454, "用户定义引用句柄标识符平化（新式）"=21747, "用户项"=3506, "有损耗元素入队列"=9130, "右泵（平面）"=3819, "右泵（阴影）"=3719, "右箭头"=3825, "右箭头值（轮廓）"=3805, "右箭头值（平面）"=3705, "右箭头值（阴影）"=21765, "右矩形值（轮廓）"=3804, "右矩形值（平面）"=3704, "右矩形值（阴影）"=21764, "右上弯管（平面）"=3814, "右上弯管（阴影）"=3714, "右下弯管（平面）"=3817, "右下弯管（阴影）"=3717, "余割"=1204, "余切"=1205, "余弦"=1201, "与"=1061, "与非"=1071, "预分配的读取二进制文件"=24135, "预览队列元素"=9112, "元电荷(C)"=23517, "元素出队列"=9113, "元素入队列"=9111, "元素同址操作结构"=2360, "圆形按钮"=3100, "圆形单选按钮"=3106, "圆形灯"=3104, "圆形开关按钮"=3118, "圆形开关按钮（性能分析）"=3112, "圆形停止按钮"=3127, "圆形指示灯（经典）"=3120, "圆形指示灯（新式）"=21012, "运动资源（程序框图常量）"=3449, "运动资源（经典）"=3448, "运动资源（新式）"=21787, "蕴含"=1080, "在后台打开变量连接"=23791, "在字符串中搜索标记"=8101, "真空光速(m/sec)"=23518, "整数拼接"=1171, "整型转换为定点"=5567, "正割"=1203, "正切"=1202, "正无穷大"=23515, "正弦"=1200, "正弦与余弦"=1220, "直接变量读取"=23785, "直接变量写入"=23788, "指示灯按钮"=3116, "指数"=1211, "制表符常量"=23502, "重力常数(Nm2/kg2)"=23519, "重排数组维数"=2055, "重组变体（警告：危险）"=2405, "重组解锁数据变量引用（警告：危险）"=2407, "重组数组"=2403, "注册会话句柄"=2319, "注册事件"=2065, "转换为64位整型"=1155, "转换为OLE变体"=8002, "转换为变体"=8201, "转换为长整型"=1142, "转换为大写字母"=1188, "转换为单精度浮点数"=1146, "转换为单精度复数"=1151, "转换为单字节整型"=1140, "转换为定点数"=5561, "转换为扩展精度浮点数"=1149, "转换为扩展精度复数"=1154, "转换为时间标识"=5560, "转换为双精度浮点数"=1147, "转换为双精度复数"=1152, "转换为双字节整型"=1141, "转换为探针字符串"=2413, "转换为特定的类"=8016, "转换为通用的类"=8017, "转换为无符号64位整型"=1156, "转换为无符号长整型"=1145, "转换为无符号单字节整型"=1143, "转换为无符号双字节整型"=1144, "转换为小写字母"=1189, "转盘（经典）"=3050, "转盘（新式）"=21732, "状态"=2198, "状态图"=2051, "准备接收"=1975, "资源索引"=1088, "子面板"=21810, "子面板（经典）"=21811, "子面板（系统）"=21823, "自动化引用句柄"=3410, "自然对数"=1209, "自然对数 (Arg +1)"=1221, "自然对数的底数"=23510, "自由标签"=2321, "字符串常量"=2007, "字符串长度"=1502, "字符串输入控件（经典）"=3200, "字符串输入控件（系统）"=21920, "字符串输入控件（新式）"=21701, "字符串数组排序"=23065, "字符串数组至路径转换"=1422, "字符串显示控件（经典）"=3201, "字符串显示控件（新式）"=21702, "字符串移位"=1536, "字符串至IP地址转换"=1711, "字符串至共享变量转换"=1830, "字符串至路径转换"=1078, "字符串至字节数组转换"=1608, "字符类"=1126, "字节流文件引用句柄"=3408, "字节数组至字符串转换"=1609, "总是复制"=2400, "组合框（经典）"=3304, "组合框（系统）"=21917, "组合框（新式）"=21604, "组合框常量"=2088, "最大值与最小值"=1108, "最近数取整"=1055, "左泵（平面）"=3813, "左泵（阴影）"=3713, "左箭头"=3826, "左矩形值（轮廓）"=3800, "左矩形值（平面）"=3700, "左矩形值（阴影）"=21760, "左上弯管（平面）"=3808, "左上弯管（阴影）"=3708, "左下弯管（平面）"=3811, "左下弯管（阴影）"=3711]
